vi "initialize.vi"(8 "error in (no error)":errorcluster, 11 "Cricket in":refnum<class "Cricket.lvclass">) -> (0 "error out":errorcluster, 3 "Cricket out":refnum<class "Cricket.lvclass">)   [LabVIEW 2017, in "Cricket.lvclass"]
uses:
  Cricket.lvclass
  ConsoleOut/Print Options.ctl
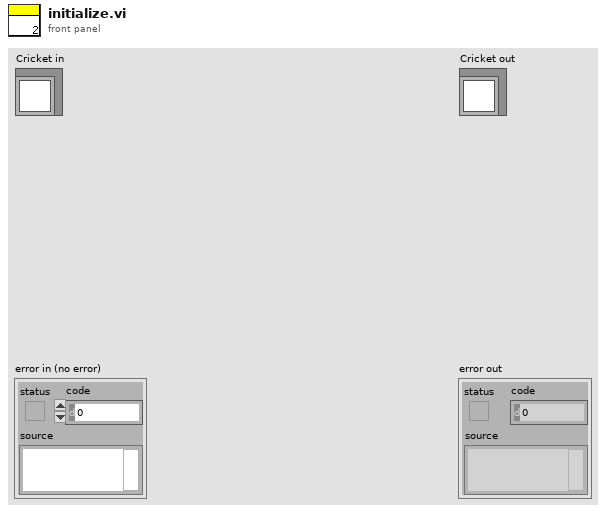
[diagram p1: front panel]
types:
  T1 = typedef "Print Options.ctl" = enum16{"Create", "Get Reference", "Print", "Print Header", "Close"}
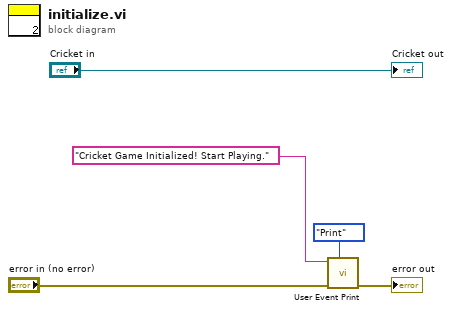
[diagram p0: block diagram]
diagram:
  n1 = call "User Event Print.vi"("Options"=Print_Options."Print", "error in (no error)"="error in (no error)", "String to Print"="Cricket Game Initialized! Start Playing." ("message")) -> ("error out"=→"error out":errorcluster)  [unwired: 7 in, 1 out]
  "Cricket out" <- "Cricket in"
